vi "Get Routes from Virtual Device.vi"(7 "error in":errorcluster, 10 "Virtual Device":string) -> (0 "error out":errorcluster, 2 "Routes":string[](array[string]), 3 "Virtual Device out":string)   [LabVIEW 2023, in "SwitchExecController.lvlib"]
uses:
  SwitchExecController.lvlib
  <vilib>/SwitchExecutive/niseCfg.llb/niseCfg Get Virtual Device.vi
  <vilib>/SwitchExecutive/niseCfg.llb/niseVirtualDevice Get Route Groups.vi
  <vilib>/SwitchExecutive/niseCfg.llb/niseRouteGroup Get Routes.vi
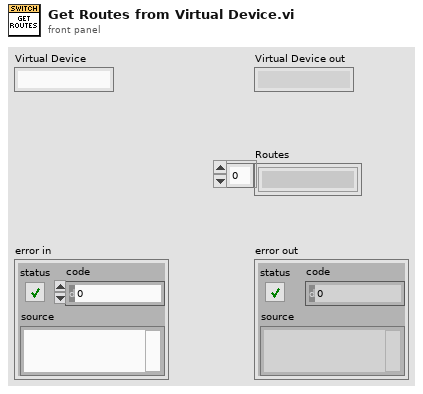
[diagram p1: front panel]
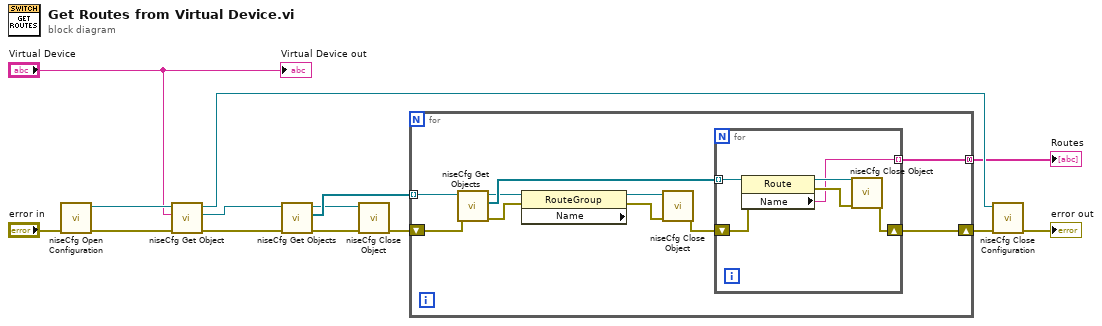
[diagram p0: block diagram]
diagram:
  n1 = call <vilib>:"niseCfg Open Configuration.vi"("error in (no error)"="error in") -> ("error out"=w11:errorcluster, "niseCfg"=w12:refnum<k7>)  [unwired: 9 in]
  n2 = call-poly <vilib>:"niseCfg Get Object.vi"("error in (no error)"=w11, "Virtual Device Name"="Virtual Device", "niseCfg"=w12) -> ("error out"=w10:errorcluster, "Virtual Device"=w3:refnum<k7>, "niseCfg out"=w4:refnum<k7>)  [unwired: 6 in]
  n3 = call-poly <vilib>:"niseCfg Get Objects.vi"("error in (no error)"=w10, "Virtual Device"=w3) -> ("error out"=w8:errorcluster, "Route Groups"=w9:refnum<k7>[], "Virtual Device out"=w6:refnum<k7>)  [unwired: 7 in]
  n4 = call <vilib>:"niseCfg Close Object.vi"("error in (no error)"=w8, "Reference"=w6) -> ("error out"=w7:errorcluster)  [unwired: 9 in]
  n5 = for {
    shift-right: [w22] -> w13
    shift-left: w7 -> [w23]
    tunnel: w9 -> [w24] mode=indexing
    tunnel: [w15] -> w2 mode=concatenating
    n6 = call-poly <vilib>:"niseCfg Get Objects.vi"("error in (no error)"=w23, "Route Group"=w24) -> ("error out"=w21:errorcluster, "Routes"=w20:refnum<k7>[], "Route Group out"=w19:refnum<k7>)  [unwired: 7 in]
    n7 = property class="RouteGroup" props=["Name"](reference=w19, error in=w21) -> (reference out=w18:refnum<k7>, error out=w17:errorcluster)  [unwired: 1 out]
    n8 = call <vilib>:"niseCfg Close Object.vi"("error in (no error)"=w17, "Reference"=w18) -> ("error out"=w16:errorcluster)  [unwired: 9 in]
    n9 = for {
      shift-right: [w26] -> w22
      shift-left: w16 -> [w29]
      tunnel: w20 -> [w30] mode=indexing
      tunnel: [w25] -> w15 mode=indexing
      n10 = property class="Route"(reference=w30, error in=w29) -> (reference out=w28:refnum<k7>, error out=w27:errorcluster, "Name"=w25:string)
      n11 = call <vilib>:"niseCfg Close Object.vi"("error in (no error)"=w27, "Reference"=w28) -> ("error out"=w26:errorcluster)  [unwired: 9 in]
    }
  }
  "Routes" <- w2
  n12 = call <vilib>:"niseCfg Close Configuration.vi"("error in (no error)"=w13, "niseCfg"=w4) -> ("error out"=→"error out":errorcluster)  [unwired: 9 in]
  "Virtual Device out" <- "Virtual Device"
